vi "userauth_publickey_fromfile.vi"() -> ()   [LabVIEW 2013]
doc: "Illustrates how to authenticate a session using public key, read from file."
uses:
  libssh2/libssh2_init_default.vi
  libssh2/libssh2_session_handshake_tcp.vi
  libssh2/libssh2.lvlib
panel:
  out "authenticated":bool
  in  "private key":path
  in  "public key":path
  in  "passphrase":string
  in  "username":string
  in  "hostname":string="localhost"
  out "error out":errorcluster
  # "This is the public key file (e.g., generated with ssh-keygen)"
  # "This is the private key file (e.g., generated with ssh-keygen)\n\nImportant: If your key files don't work, try generating keys\nwith the following command: \"ssh-keygen -m PEM -t rsa\".\nThis will create a key file with the header\n\"-----BEGIN RSA PRIVATE KEY-----\" as is expected by libssh2."
  # "This is the passphrase for your private key."
  # "When everything goes right, this status should be TRUE."
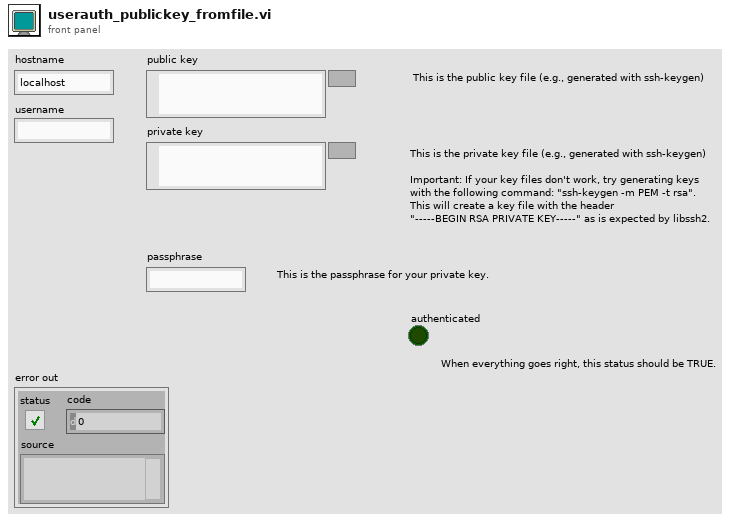
[diagram p1: front panel]
types:
  T1 = typedef "libssh2.lvlib/Session Refnum.ctl" = refnum<k1>
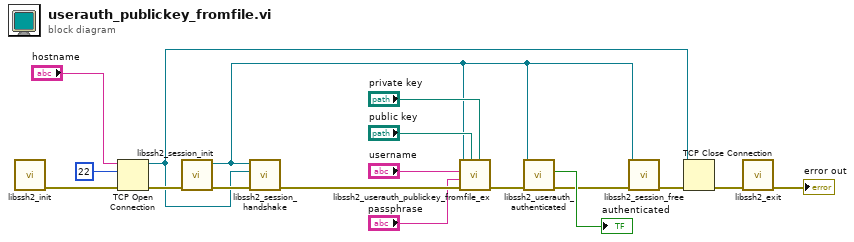
[diagram p0: block diagram]
diagram:
  n1 = call-poly "libssh2_init.vi"() -> ("error out"=w18:errorcluster)  [unwired: 11 in]
  n2 = TCP Open Connection(address="hostname", remote port or service name=u16 22, error in (no error)=w18) -> (connection ID=w9:refnum<k5>, error out=w10:errorcluster)  [unwired: 2 in]
  n3 = call "libssh2_session_init.vi"("error in (no error)"=w10) -> ("error out"=w13:errorcluster, "session"=w2:T1)  [unwired: 9 in]
  n4 = call-poly "libssh2_session_handshake.vi"("error in (no error)"=w13, "tcp connection"=w9, "session"=w2) -> ("error out"=w8:errorcluster)  [unwired: 8 in]
  n5 = call "libssh2_userauth_publickey_fromfile_ex.vi"("private key"="private key", "public key"="public key", "error in (no error)"=w8, "passphrase"="passphrase", "username"="username", "session"=w2) -> ("error out"=w7:errorcluster)  [unwired: 5 in]
  n6 = call "libssh2_userauth_authenticated.vi"("error in (no error)"=w7, "session"=w2) -> ("error out"=w1:errorcluster, "authenticated"=→"authenticated":bool)  [unwired: 8 in]
  n7 = call "libssh2_session_free.vi"("error in (no error)"=w1, "session"=w2) -> ("error out"=w11:errorcluster)  [unwired: 9 in]
  n8 = TCP Close Connection(connection ID=w9, error in (no error)=w11) -> (error out=w15:errorcluster)  [unwired: 1 in, 1 out]
  n9 = call "libssh2_exit.vi"("error in (no error)"=w15) -> ("error out"=→"error out":errorcluster)  [unwired: 10 in]
